vi "UDP FGV.vi"(7 "Action":T1, 8 "error in (no error)":errorcluster, 9 "Port":u16, 10 "IP Address":string, 11 "connection ID":refnum<k16>) -> (0 "error out":errorcluster, 1 "Port Out":u16, 2 "IP Address out":string, 3 "connection ID out":refnum<k16>)   [LabVIEW 2014]
doc: "Functional Global Variable used to maintain all outgoing UDP connection settings."
uses:
  Controls/UDP Reference Action Enum.ctl
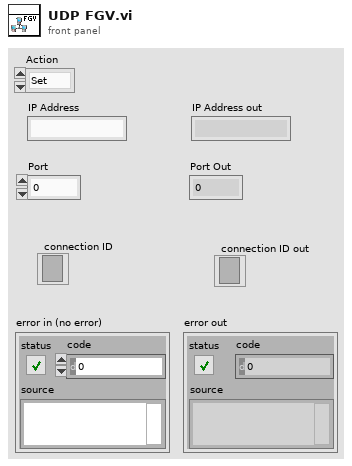
[diagram p1: front panel]
types:
  T1 = typedef "UDP Reference Action Enum.ctl" = enum16{"Set", "Get"}
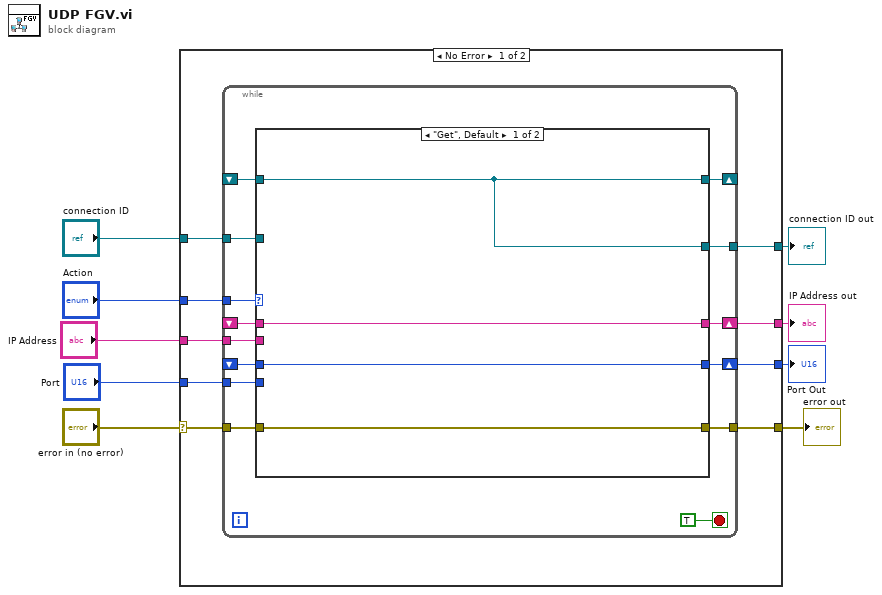
[diagram p0: block diagram]
diagram:
  n1 = case shown="No Error" "error in (no error)" {
    selector: "error in (no error)" -> [w16 w43]
    tunnel: "Action" -> [w18 _]
    tunnel: "connection ID" -> [w17 w44]
    tunnel: [w15 w44] -> w6
    tunnel: [w14 w43] -> w5
    tunnel: "IP Address" -> [w13 w42]
    tunnel: [w12 w42] -> w3
    tunnel: "Port" -> [w11 w41]
    tunnel: [w10 w41] -> w1
    frame No Error {
      n2 = while {
        tunnel: w18 -> [w31]
        tunnel: w17 -> [w30]
        tunnel: w16 -> [w29]
        shift-right: [w28] -> _
        shift-left: _ -> [w27]
        tunnel: [w26] -> w15
        tunnel: [w25] -> w14
        tunnel: w13 -> [w24]
        shift-right: [w23] -> w12
        shift-left: _ -> [w22]
        tunnel: w11 -> [w21]
        shift-right: [w20] -> w10
        shift-left: _ -> [w19]
        stop <- TRUE stop-if-true
        n3 = case shown="\"Get\", Default" w31 {
          tunnel: w30 -> [_ w40]
          tunnel: w29 -> [w35 w39]
          tunnel: [w36 w40] -> w28
          tunnel: w27 -> [w36 _]
          tunnel: [w36 w40] -> w26
          tunnel: [w35 w39] -> w25
          tunnel: w24 -> [_ w38]
          tunnel: [w34 w38] -> w23
          tunnel: w22 -> [w34 _]
          tunnel: w21 -> [_ w37]
          tunnel: [w33 w37] -> w20
          tunnel: w19 -> [w33 _]
          frame "Get", Default {
          }
          frame "Set" {
          }
        }
      }
    }
    frame Error {
    }
  }
  "error out" <- w5
  "connection ID out" <- w6
  "IP Address out" <- w3
  "Port Out" <- w1
